vi "Read.vi"(0 "TDCManager":T1, 5 "Buffer (10000 entries)":i32[](array[numeric])=array[10001 elements], 11 "error in (no error)":errorcluster) -> (4 "TDCManager":T1, 6 "TDC hit times":i32[](array[numeric]), 8 "Hits":i32, 10 "Words read":i32, 15 "error out":errorcluster)   [LabVIEW 2016, in "HPTDC Driver Library.lvlib"]
uses:
  HPTDC Driver Library.lvlib
  Typedefs/TDCManager.ctl
  C:/Users/CRT Controller/CRTC Labview Application/Source/HPTDC Driver Library Folder/Library files/hptdc_net4_3.7.0_x64.dll
  hptdc_net4_3.7.0_x64.dll
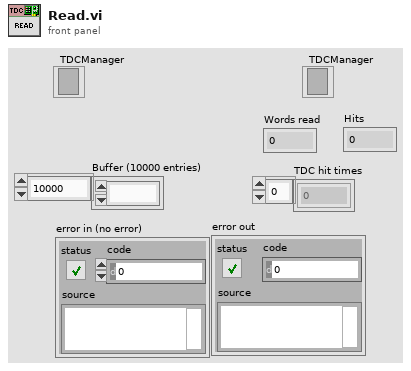
[diagram p1: front panel]
types:
  T1 = typedef "HPTDC Driver Library.lvlib/TDCManager.ctl" = refnum<k24>
  T2 = typedef "Semaphore RefNum" = refnum<k1>
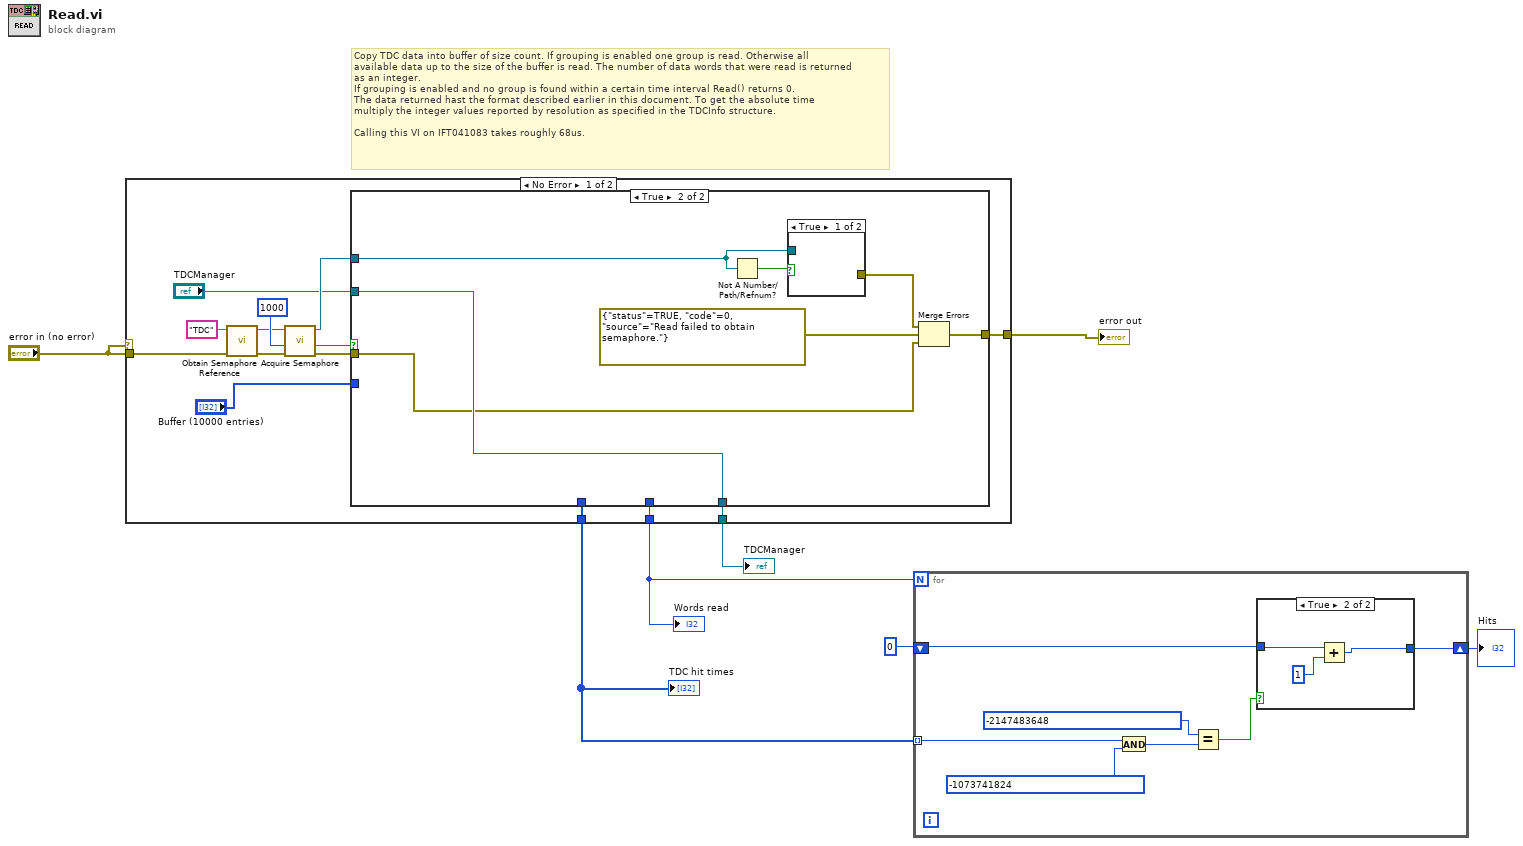
[diagram p0: block diagram]
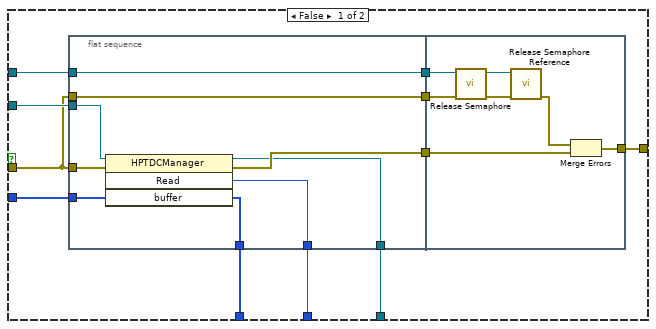
[diagram p2: hidden frame]
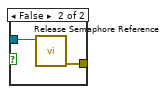
[diagram p3: hidden frame]
diagram:
  # "Copy TDC data into buffer of size count. If grouping is enabled one group is read. Otherwise all\navailable data up to the size of the buffer is read. The number of data words that were read is returned\nas an integer.\nIf grouping is enabled and no group is found within a certain time interval Read() returns 0.\nThe data returned hast the format described earlier in this document. To get the absolute time\nmultiply the integer values reported by resolution as specified in the TDCInfo structure.\n\nCalling this VI on IFT041083 takes roughly 68us."
  n1 = case shown="No Error" "error in (no error)" {
    tunnel: [w13 _] -> w7
    tunnel: [w12 w58] -> w6
    tunnel: "error in (no error)" -> [w10 w58]
    tunnel: [w9 _] -> w5
    tunnel: [w8 _] -> w2
    frame No Error {
      n2 = call <vilib>:"Obtain Semaphore Reference.vi"("error in (no error)"=w10, "name (unnamed)"="TDC") -> ("error out"=w19:errorcluster, "semaphore"=w20:T2)  [unwired: 3 in, 1 out]
      n3 = call <vilib>:"Acquire Semaphore.vi"("error in (no error)"=w19, "ms timeout (-1)"=1000, "semaphore"=w20) -> ("error out"=w16:errorcluster, "timed out"=w17:bool, "semaphore out"=w15:T2)  [unwired: 2 in]
      n4 = case shown="True" w17 {
        tunnel: "TDCManager" -> [w32 w55]
        tunnel: w16 -> [w29 w49]
        tunnel: w15 -> [w27 w51]
        tunnel: [w26 w55] -> w13
        tunnel: [w25 w53] -> w12
        tunnel: [w24 _] -> w8
        tunnel: "Buffer (10000 entries)" -> [w23 _]
        tunnel: [w22 _] -> w9
        frame False {
          n5 = flat-sequence {
            tunnel: w29 -> [w41]
            tunnel: w32 -> [w40]
            tunnel: [w39] -> w31
            tunnel: w29 -> [w38]
            tunnel: [w38] -> w30
            tunnel: [w37] -> w28
            tunnel: w27 -> [w37]
            tunnel: [w36] -> w26
            tunnel: [w35] -> w24
            tunnel: w23 -> [w34]
            tunnel: [w33] -> w22
            tunnel: w31 -> [w48]
            tunnel: w30 -> [w45]
            tunnel: w28 -> [w43]
            tunnel: [w42] -> w25
            frame #0 {
              n6 = invoke class="HPTDCManager" method="Read"(reference=w40, error in=w41, "buffer"=w34) -> (reference out=w36:T1, error out=w39:errorcluster, "Read"=w35:i32, "buffer"=w33:i32[])  [unwired: 1 in]
            }
            frame #1 {
              n7 = call <vilib>:"Release Semaphore.vi"("error in (no error)"=w45, "semaphore"=w43) -> ("error out"=w46:errorcluster, "semaphore out"=w47:T2)  [unwired: 4 in]
              n8 = call <vilib>:"Release Semaphore Reference.vi"("error in (no error)"=w46, "semaphore"=w47) -> ("error out"=w44:errorcluster)  [unwired: 8 in, 1 out]
              n9 = Merge Errors(w44, w48) -> (w42:errorcluster)
            }
          }
        }
        frame True {
          n10 = Not A Number/Path/Refnum?(number/path/refnum=w51) -> (NaN/Path/Refnum?=w50:bool)
          n11 = case shown="True" w50 {
            tunnel: [_ w57] -> w52
            tunnel: w51 -> [_ w56]
            frame True {
            }
            frame False {
              n12 = call <vilib>:"Release Semaphore Reference.vi"("semaphore"=w56) -> ("error out"=w57:errorcluster)  [unwired: 9 in, 1 out]
            }
          }
          n13 = Merge Errors(w52, errorcluster {"status"=TRUE, "code"=0, "source"="Read failed to obtain semaphore."} ("error out"), w49) -> (w53:errorcluster)
        }
      }
    }
    frame Error {
    }
  }
  "error out" <- w6
  "TDCManager" <- w7
  "TDC hit times" <- w5
  "Words read" <- w2
  n14 = for {
    N: w2 -> [_]
    tunnel: w5 -> [w65] mode=indexing
    shift-right: [w59] -> w3
    shift-left: 0 -> [w60]
    n15 = And(x=w65, y=-1073741824) -> (x .and. y?=w63:i32)
    n16 = Equal?(x=-2147483648 ("y"), y=w63) -> (x = y?=w61:bool)
    n17 = case shown="True" w61 {
      tunnel: w60 -> [w66 w69]
      tunnel: [w66 w68] -> w59
      frame False {
      }
      frame True {
        n18 = Add(x=w69, y=1) -> (x+y=w68:i32)
      }
    }
  }
  "Hits" <- w3
